vi "sub vi all info.vi"   [LabVIEW 2019]
uses:
  <vilib>/httpClient/POSTBuffer.vi
  <vilib>/httpClient/LabVIEWHTTPClient.lvlib
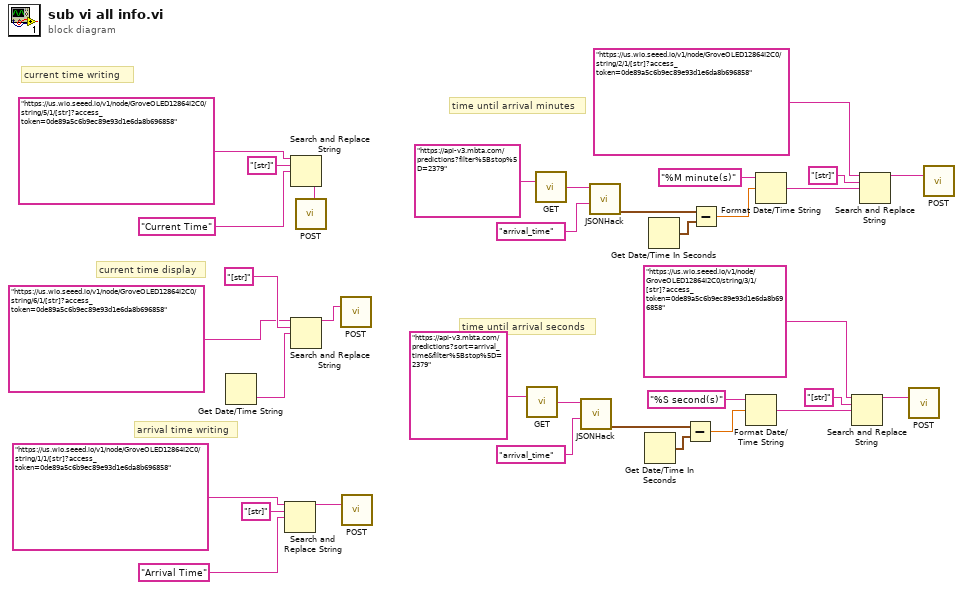
[diagram p0: block diagram]
diagram:
  # "arrival time writing"
  # "time until arrival seconds"
  # "time until arrival minutes"
  # "current time display"
  # "current time writing"
  n1 = Get Date/Time String() -> (time string=w1:string)  [unwired: 3 in, 1 out]
  n2 = Search and Replace String(input string="https://us.wio.seeed.io/v1/node/GroveOLED12864I2C0/string/1/1/[str]?access_token=0de89a5c6b9ec89e93d1e6da8b696858", search string="[str]", replace string="Arrival Time" ("replace string (\"\")")) -> (result string=w5:string)  [unwired: 5 in, 3 out]
  n3 = Search and Replace String(input string="https://us.wio.seeed.io/v1/node/GroveOLED12864I2C0/string/5/1/[str]?access_token=0de89a5c6b9ec89e93d1e6da8b696858", search string="[str]", replace string="Current Time" ("replace string (\"\")")) -> (result string=w33:string)  [unwired: 5 in, 3 out]
  n4 = Search and Replace String(input string="https://us.wio.seeed.io/v1/node/GroveOLED12864I2C0/string/6/1/[str]?access_token=0de89a5c6b9ec89e93d1e6da8b696858", search string="[str]", replace string=w1) -> (result string=w29:string)  [unwired: 5 in, 3 out]
  n5 = call-poly <vilib>:"POST.vi"("url"=w33) -> ()  [unwired: 11 in, 4 out]
  n6 = call-poly <vilib>:"POST.vi"("url"=w29) -> ()  [unwired: 11 in, 4 out]
  n7 = call-poly <vilib>:"POST.vi"("url"=w5) -> ()  [unwired: 11 in, 4 out]
  n8 = call <vilib>:"GET.vi"("url"="https://api-v3.mbta.com/predictions?sort=arrival_time&filter%5Bstop%5D=2379") -> ("body"=w16:string)  [unwired: 11 in, 3 out]
  n9 = call <vilib>:"GET.vi"("url"="https://api-v3.mbta.com/predictions?filter%5Bstop%5D=2379") -> ("body"=w27:string)  [unwired: 11 in, 3 out]
  n10 = call "JSONHack.vi"("search name"="arrival_time", "JSON in"=w16) -> ("Property (time stamp)"=w17:timestamp)  [unwired: 6 in, 3 out]
  n11 = call "JSONHack.vi"("search name"="arrival_time", "JSON in"=w27) -> ("Property (time stamp)"=w28:timestamp)  [unwired: 6 in, 3 out]
  n12 = Get Date/Time In Seconds() -> (seconds since 1Jan1904=w15:timestamp)
  n13 = Get Date/Time In Seconds() -> (seconds since 1Jan1904=w26:timestamp)
  n14 = Subtract(x=w17, y=w15) -> (x-y=w14:dbl)
  n15 = Subtract(x=w28, y=w26) -> (x-y=w25:dbl)
  n16 = Format Date/Time String(time format string (%c)="%S second(s)", seconds (now)=w14) -> (date/time string=w10:string)  [unwired: 1 in]
  n17 = Format Date/Time String(time format string (%c)="%M minute(s)", seconds (now)=w25) -> (date/time string=w21:string)  [unwired: 1 in]
  n18 = Search and Replace String(input string="https://us.wio.seeed.io/v1/node/GroveOLED12864I2C0/string/3/1/[str]?access_token=0de89a5c6b9ec89e93d1e6da8b696858", search string="[str]", replace string=w10) -> (result string=w8:string)  [unwired: 5 in, 3 out]
  n19 = Search and Replace String(input string="https://us.wio.seeed.io/v1/node/GroveOLED12864I2C0/string/2/1/[str]?access_token=0de89a5c6b9ec89e93d1e6da8b696858", search string="[str]", replace string=w21) -> (result string=w19:string)  [unwired: 5 in, 3 out]
  n20 = call-poly <vilib>:"POST.vi"("url"=w8) -> ()  [unwired: 11 in, 4 out]
  n21 = call-poly <vilib>:"POST.vi"("url"=w19) -> ()  [unwired: 11 in, 4 out]
